vi "ConfigureDlg.vi"(8 "error in (no error)":errorcluster, 11 "SiemensDigitalEnergyMeter in":refnum<class "SiemensDigitalEnergyMeter.lvclass">) -> (0 "error out":errorcluster, 2 "Changed":bool, 3 "SiemensDigitalEnergyMeter out":refnum<class "SiemensDigitalEnergyMeter.lvclass">)   [LabVIEW 2018, in "SensorPlugins.lvlib" / "SiemensDigitalEnergyMeter.lvclass"]
doc: "This VI creates allow the user to configure the instrument using the provided panel and saves the instruments configuration to file, a new file or cancels the entire operation."
uses:
  SiemensDigitalEnergyMeter.lvclass
  C:/Program Files (x86)/National Instruments/LabVIEW 2018/user.lib/NIST/BaseClasses/BasePlugin_class/BasePlugin.lvclass
  TypeDefinitions/SiemensDigitalEnergyMeterControls.ctl
  TypeDefinitions/MeasurementControls.ctl
  <userlib>/NIST/BaseClasses/BasePlugin_class/BasePlugin.lvclass/BasePlugin.ctl
  <userlib>/NIST/BaseClasses/BasePlugin_class/Accessors/Read PluginIniFilePath.vi
  <userlib>/NIST/BaseClasses/BasePlugin_class/Accessors/Write PluginIniFilePath.vi
  <vilib>/Utility/config.llb/NI_LVConfig.lvlib
panel:
  in  "MeasurementCluster":T1
  in  "Siemens Digital Energy Meter":T2 {"Measurement(s)" items=["kWh System"=4000, "kVARh System"=4007, "kVAh System"=4010, "kVA System"=4012, "Volts L1 to L2"=4018, "Volts L2 to L3"=4019, "Volts L1 to L2"=4020, "Line Frequency"=4021, "kW L1"=4028, "kW L2"=4029, "kW L3"=4030, "kVAR L1"=4037, "kVAR L2"=4038, "kVAR L3"=4039, "kVA L1"=4046, "kVA L2"=4047, "kVA L3"=4048, "Apparent PF L1"=4052, "Apparent PF L2"=4053, "Apparent PF L3"=4054, "Amps L1"=4055, "Amps L2"=4056, "Amps L3"=4057, "Volts L1 to Neutral"=4058, "Volts L2 to Neutral"=4059, "Volts L3 to Neutral"=4060, "Firmware Major Revision"=4068, "Firmware Minor Revision "=4069, "Model Number "=4200, "Serial Number"=4205, "Hardware ID"=4510]}
  in  "btnSaveAs":bool
  in  "btnSave":bool
  in  "btnCancel":bool
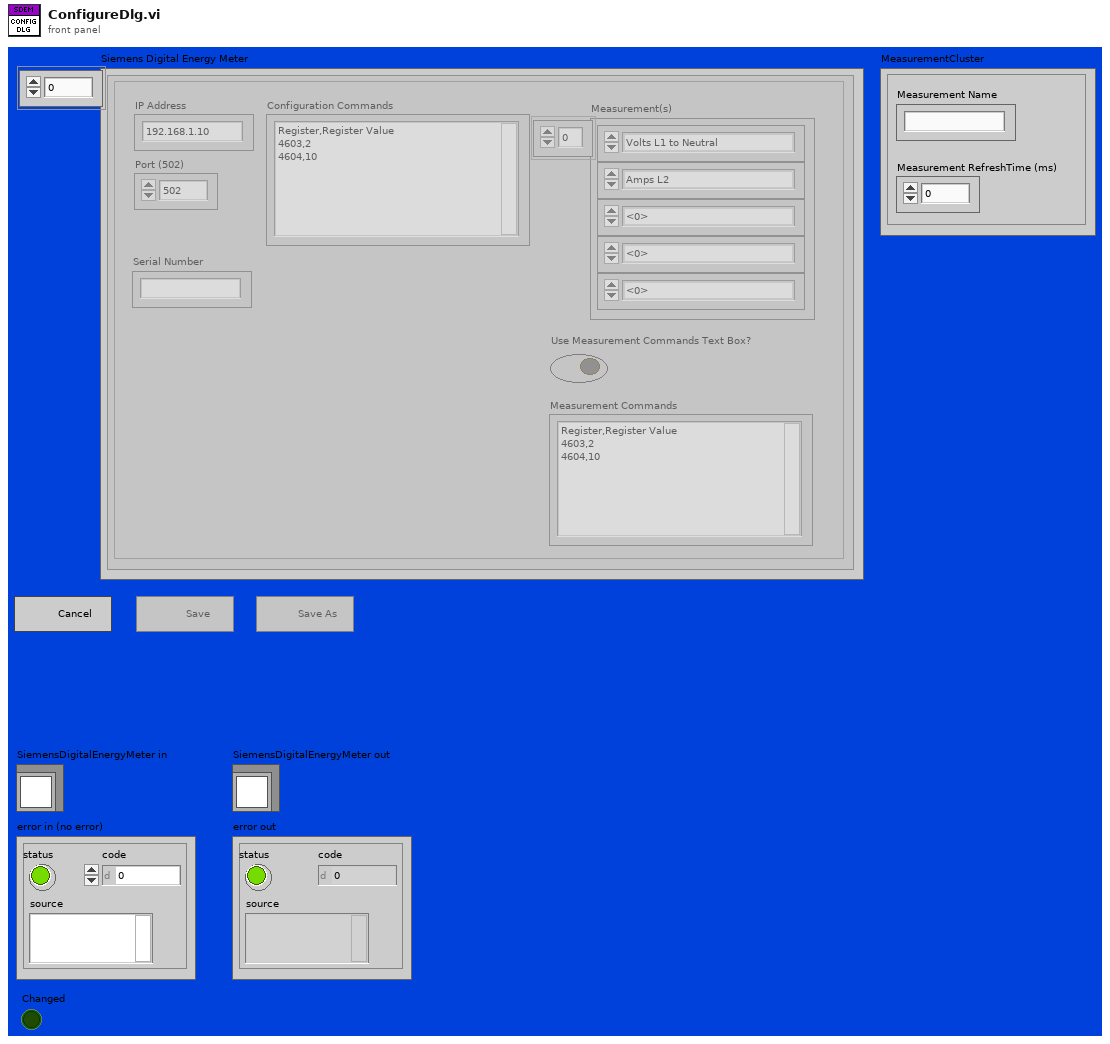
[diagram p1: front panel]
types:
  T1 = typedef "SensorPlugins.lvlib/SiemensDigitalEnergyMeter.lvclass/MeasurementControls.ctl" = cluster{"Measurement RefreshTime (ms)":u32, "Measurement Name":string}
  T2 = typedef "SensorPlugins.lvlib/SiemensDigitalEnergyMeter.lvclass/SiemensDigitalEnergyMeterControls.ctl" = cluster{"Measurement(s)":u16[], "IP Address":string, "Port (502)":u16, "Configuration Commands":string, "Use Measurement Commands Text Box?":bool, "Measurement Commands":string, "Connected?":bool, "Serial Number":string}[]
  T3 = enum32{"Invalid", "Default", "Floating", "Floating/Auto-Hide", "Modal"}
  T4 = enum32{"Invalid", "Standard", "Closed", "Hidden", "Minimized", "Maximized"}
  T5 = enum8{"Enabled", "Disabled", "Disabled and Grayed Out"}
  T6 = cluster{"Measurement(s)":u16[], "IP Address":string, "Port (502)":u16, "Configuration Commands":string, "Use Measurement Commands Text Box?":bool, "Measurement Commands":string, "Connected?":bool, "Serial Number":string}
  T7 = typedef "NI_LVConfig.lvlib/Config Data RefNum.ctl" = refnum<k1>
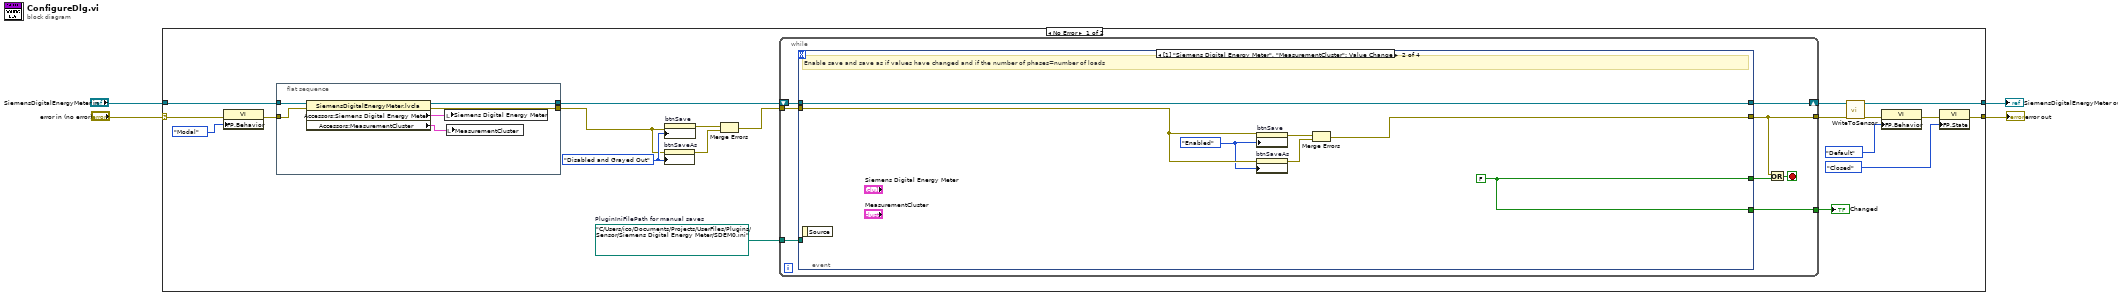
[diagram p0: block diagram]
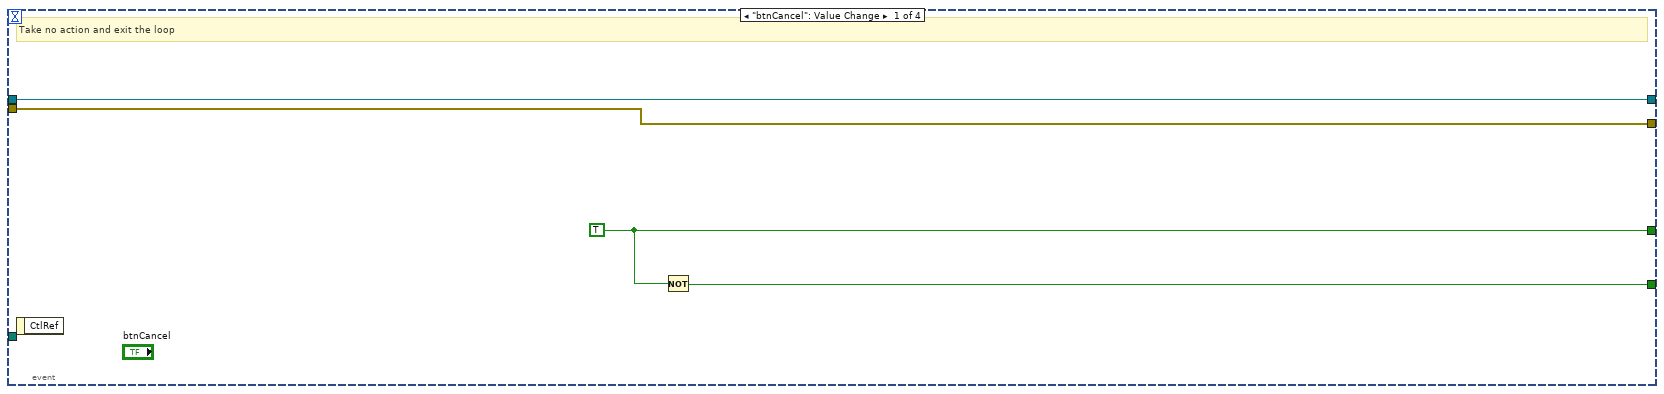
[diagram p2: hidden frame]
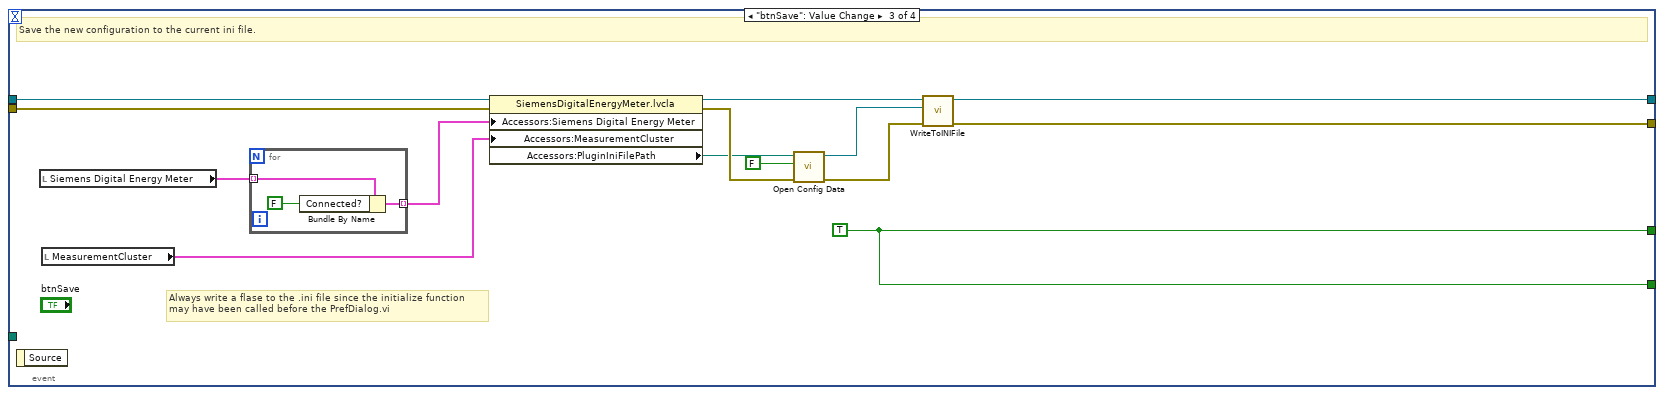
[diagram p3: hidden frame]
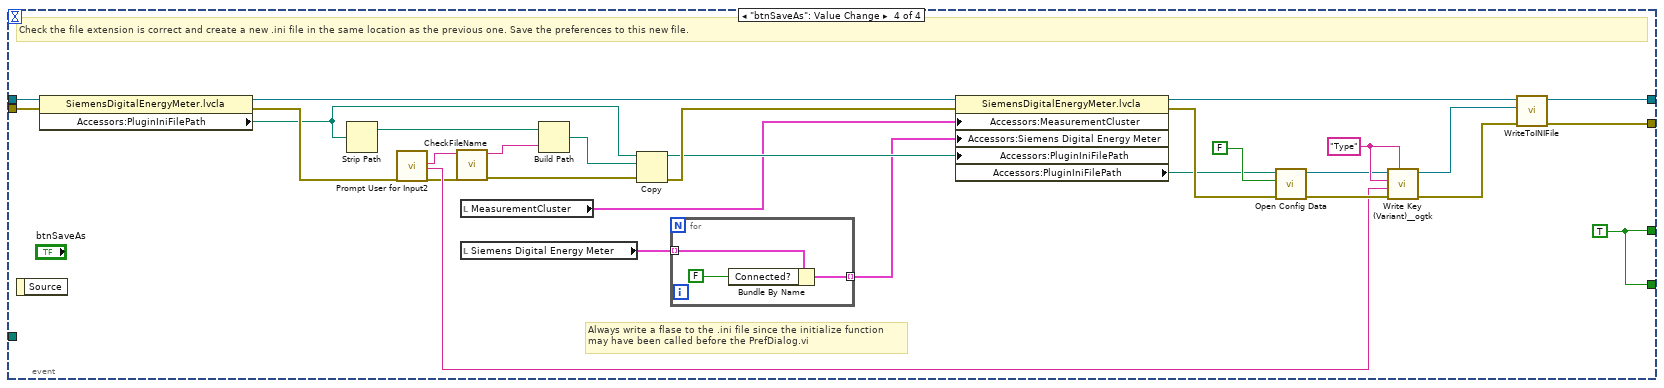
[diagram p4: hidden frame]
diagram:
  n1 = case shown="No Error" "error in (no error)" {
    selector: "error in (no error)" -> [w19 w99]
    tunnel: [w5 w100] -> w1
    tunnel: [w21 w99] -> w2
    tunnel: "SiemensDigitalEnergyMeter in" -> [w20 w100]
    frame No Error {
      w12 = T5."Disabled and Grayed Out" ("Disabled")
      w9 = path "C:/Users/ico/Documents/Projects/UserFiles/Plugins/Sensor/Siemens Digital Energy Meter/SDEM0.ini"  # PluginIniFilePath for manual saves
      n2 = property class="VI"(error in=w19, "FP.Behavior"=T3."Modal" ("Front Panel Window:Behavior")) -> (error out=w17:errorcluster)  [unwired: 1 in, 1 out]
      n3 = flat-sequence {
        tunnel: w20 -> [w29]
        tunnel: [w27] -> w16
        tunnel: [w26] -> w11
        tunnel: w17 -> [w30]
        frame #0 {
          n4 = property class="SiemensDigitalEnergyMeter.lvcla"(reference=w29, error in=w30) -> (reference out=w27:refnum<class "SiemensDigitalEnergyMeter.lvclass">, error out=w26:errorcluster, "Accessors:Siemens Digital Energy Meter"=w28:T2, "Accessors:MeasurementCluster"=w25:T1)
          n5 = local write "Siemens Digital Energy Meter"(w28) -> ()
          n6 = local write "MeasurementCluster"(w25) -> ()
        }
      }
      n7 = property on="btnSaveAs" class="Bool"(error in=w11, "DisabledEnum"=w12) -> (error out=w13:errorcluster)  [unwired: 1 in, 1 out]
      n8 = property on="btnSave" class="Bool"(error in=w11, "DisabledEnum"=w12) -> (error out=w14:errorcluster)  [unwired: 1 in, 1 out]
      n9 = Merge Errors(w14, w13) -> (w10:errorcluster)
      n10 = while {
        shift-right: [w37] -> w8
        shift-left: w16 -> [w38]
        tunnel: w10 -> [w36]
        tunnel: [w33] -> w7
        tunnel: [w35] -> w15
        tunnel: w9 -> [w31]
        stop <- w34 stop-if-true
        n11 = event shown="[1] \"Siemens Digital Energy Meter\", \"MeasurementCluster\": Value Change" {
          selector: _ -> [_ _ _ _]
          dyn-events: _ -> [_ _ _ _]
          timeout: _ -> [_ _ _ _]
          tunnel: w38 -> [w42 w46 w60 w78]
          tunnel: [w40 w49 w62 w94] -> w32
          tunnel: [w42 w46 w58 w91] -> w37
          tunnel: w36 -> [w41 w48 w52 w77]
          tunnel: [w41 w47 w54 w89] -> w33
          tunnel: [w39 w49 w62 w94] -> w35
          tunnel: w31 -> [_ _ _ _]
          event "btnCancel": Value Change {
            w40 = TRUE
            # "Take no action and exit the loop"
            n12 = event-data() -> ()  [unwired: 1 in, 1 out]
            n13 = Not(x=w40) -> (.not. x?=w39:bool)
          }
          event Value Change {
            w43 = T5."Enabled" ("Disabled")
            w49 = FALSE
            # "Enable save and save as if values have changed and if the number of phases=number of loads"
            n14 = event-data() -> ()  [unwired: 1 in, 1 out]
            n15 = property on="btnSaveAs" class="Bool"(error in=w48, "DisabledEnum"=w43) -> (error out=w45:errorcluster)  [unwired: 1 in, 1 out]
            n16 = property on="btnSave" class="Bool"(error in=w48, "DisabledEnum"=w43) -> (error out=w44:errorcluster)  [unwired: 1 in, 1 out]
            n17 = Merge Errors(w44, w45) -> (w47:errorcluster)
          }
          event "btnSave": Value Change {
            w62 = TRUE
            # "Always write a flase to the .ini file since the initialize function\nmay have been called before the PrefDialog.vi"
            # "Save the new configuration to the current ini file."
            n18 = event-data() -> ()  [unwired: 1 in, 1 out]
            n19 = local read "Siemens Digital Energy Meter"() -> (w61:T2)
            n20 = local read "MeasurementCluster"() -> (w50:T1)
            n21 = for {
              tunnel: w61 -> [w65] mode=indexing
              tunnel: [w66] -> w53 mode=indexing
              n22 = Bundle By Name(cluster=w65, "Connected?"=FALSE) -> (w66:T6)
            }
            n23 = property class="SiemensDigitalEnergyMeter.lvcla"(reference=w60, error in=w52, "Accessors:Siemens Digital Energy Meter"=w53, "Accessors:MeasurementCluster"=w50) -> (reference out=w59:refnum<class "SiemensDigitalEnergyMeter.lvclass">, error out=w55:errorcluster, "Accessors:PluginIniFilePath"=w51:path)
            n24 = call <vilib>:"Open Config Data.vi"("error in (no error)"=w55, "create file if necessary (T)"=FALSE, "configuration file path"=w51) -> ("error out"=w56:errorcluster, "refnum"=w57:T7)  [unwired: 6 in, 1 out]
            n25 = call-dynamic "WriteToINIFile.vi"("error in (no error)"=w56, "Refnum in"=w57, "SiemensDigitalEnergyMeter in"=w59) -> ("error out"=w54:errorcluster, "SiemensDigitalEnergyMeter out"=w58:refnum<class "SiemensDigitalEnergyMeter.lvclass">)  [unwired: 7 in]
          }
          event "btnSaveAs": Value Change {
            w88 = "Type" ("section (optional)")
            w94 = TRUE
            # "Always write a flase to the .ini file since the initialize function\nmay have been called before the PrefDialog.vi"
            # "Check the file extension is correct and create a new .ini file in the same location as the previous one. Save the preferences to this new file."
            n26 = event-data() -> ()  [unwired: 1 in, 1 out]
            n27 = property class="SiemensDigitalEnergyMeter.lvcla"(reference=w78, error in=w77) -> (reference out=w76:refnum<class "SiemensDigitalEnergyMeter.lvclass">, error out=w75:errorcluster, "Accessors:PluginIniFilePath"=w74:path)
            n28 = Strip Path(path=w74) -> (stripped path=w83:path)  [unwired: 1 out]
            n29 = call "Prompt User for Input2"("error in (no error)"=w75) -> ("File Name"=w69:string, "PluginType"=w72:string, "error out"=w68:errorcluster)  [unwired: 15 in, 1 out]
            n30 = call "CheckFileName.vi"("Error In"=w68, "File Name in"=w69) -> ("Error Out"=w70:errorcluster, "File Name out"=w71:string)  [unwired: 8 in]
            n31 = local read "MeasurementCluster"() -> (w67:T1)
            n32 = local read "Siemens Digital Energy Meter"() -> (w93:T2)
            n33 = Build Path(base path=w83, name or relative path=w71) -> (appended path=w82:path)
            n34 = Copy(8:w70, 10:w82, 11:w74) -> (0:w81:errorcluster, 3:w79:path)  [unwired: 2 in, 1 out]
            n35 = for {
              tunnel: w93 -> [w97] mode=indexing
              tunnel: [w98] -> w73 mode=indexing
              n36 = Bundle By Name(cluster=w97, "Connected?"=FALSE) -> (w98:T6)
            }
            n37 = property class="SiemensDigitalEnergyMeter.lvcla"(reference=w76, error in=w81, "Accessors:MeasurementCluster"=w67, "Accessors:Siemens Digital Energy Meter"=w73, "Accessors:PluginIniFilePath"=w79) -> (reference out=w92:refnum<class "SiemensDigitalEnergyMeter.lvclass">, error out=w90:errorcluster, "Accessors:PluginIniFilePath"=w80:path)
            n38 = call <vilib>:"Open Config Data.vi"("error in (no error)"=w90, "create file if necessary (T)"=FALSE, "configuration file path"=w80) -> ("error out"=w86:errorcluster, "refnum"=w87:T7)  [unwired: 6 in, 1 out]
            n39 = call <userlib>:"Write Key (Variant)__ogtk.vi"("section"=w88, "error in (no error)"=w86, "key-value"=w72, "key (optional)"=w88, "refnum"=w87) -> ("error out"=w85:errorcluster, "refnum out"=w84:T7)  [unwired: 5 in]
            n40 = call-dynamic "WriteToINIFile.vi"("error in (no error)"=w85, "Refnum in"=w84, "SiemensDigitalEnergyMeter in"=w92) -> ("error out"=w89:errorcluster, "SiemensDigitalEnergyMeter out"=w91:refnum<class "SiemensDigitalEnergyMeter.lvclass">)  [unwired: 7 in]
          }
        }
        n41 = Or(x=w33, y=w32) -> (x .or. y?=w34:bool)
      }
      "Changed" <- w15
      n42 = call-dynamic "WriteToSensor.vi"("error in (no error)"=w7, "SiemensDigitalEnergyMeter in"=w8) -> ("error out"=w6:errorcluster, "SiemensDigitalEnergyMeter out"=w5:refnum<class "SiemensDigitalEnergyMeter.lvclass">)  [unwired: 8 in]
      n43 = property class="VI"(error in=w6, "FP.Behavior"=T3."Default" ("Front Panel Window:Behavior")) -> (error out=w24:errorcluster)  [unwired: 1 in, 1 out]
      n44 = property class="VI"(error in=w24, "FP.State"=T4."Closed" ("Front Panel Window:State")) -> (error out=w21:errorcluster)  [unwired: 1 in, 1 out]
    }
    frame Error {
    }
  }
  "error out" <- w2
  "SiemensDigitalEnergyMeter out" <- w1
